vi "save_config.vi"   [LabVIEW 2011]
doc: "Illustrates how to create and write a configuration settings file.\n\nInstructions:\nEnter values in the controls on the front panel then click on the Run Arrow.\nTo read the file, run Read Configuration Settings File.vi located in the file\\config.llb."
uses:
  global.vi
  <vilib>/Utility/config.llb/Write Key (I32).vi
  <vilib>/Utility/config.llb/Write Key (Boolean).vi
  <vilib>/Utility/config.llb/Write Key (Double).vi
  <vilib>/Utility/config.llb/Write Key (String).vi
  <vilib>/Utility/config.llb/NI_LVConfig.lvlib
types:
  T1 = typedef "NI_LVConfig.lvlib/Config Data RefNum.ctl" = refnum<k1>
  T2 = typedef "scale.ctl" = dbl
  T3 = typedef "sampling_rate.ctl" = ext
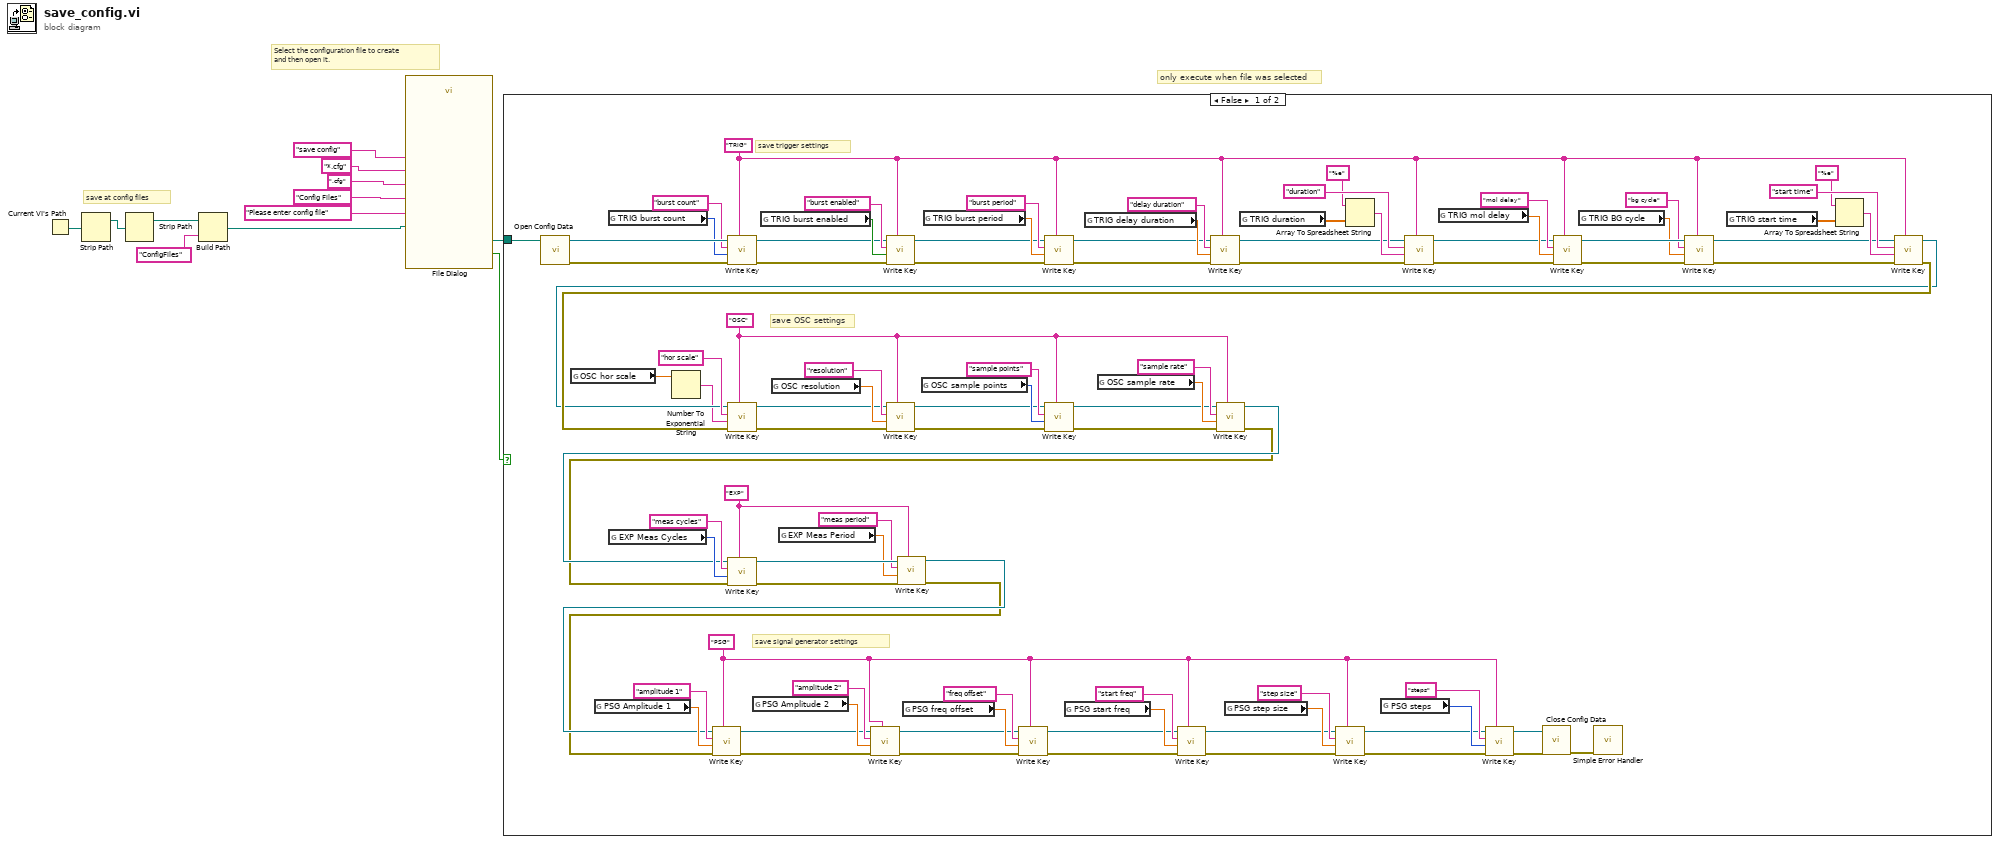
[diagram p0: block diagram]
diagram:
  # "only execute when file was selected"
  # "save at config files"
  # "Select the configuration file to create\nand then open it."
  n1 = Current VI's Path() -> (path=w6:path)
  n2 = Strip Path(path=w6) -> (stripped path=w3:path)  [unwired: 1 out]
  n3 = Strip Path(path=w3) -> (stripped path=w2:path)  [unwired: 1 out]
  n4 = Build Path(base path=w2, name or relative path="ConfigFiles") -> (appended path=w4:path)
  n5 = call "File Dialog"("start path"=w4, "prompt"="Please enter config file", "button label"="save config", "default name"=".cfg", "pattern (all files)"="*.cfg", "pattern label"="Config Files") -> ("selected path"=w12:path, "cancelled"=w1:bool)  [unwired: 6 in, 2 out]
  n6 = case shown="False" w1 {
    tunnel: w12 -> [w101 _]
    frame False {
      w28 = "PSG"
      w19 = "EXP"
      w57 = "OSC"
      w15 = "TRIG"
      # "save signal generator settings"
      # "save OSC settings"
      # "save trigger settings"
      n7 = call <vilib>:"Open Config Data.vi"("configuration file path"=w101) -> ("error out"=w104:errorcluster, "refnum"=w105:T1)  [unwired: 2 in, 7 out]
      n8 = global read "global.vi" "OSC hor scale"() -> (w27:T2)
      n9 = global read "global.vi" "PSG Amplitude 1"() -> (w38:dbl)
      n10 = global read "global.vi" "TRIG burst count"() -> (w100:i32)
      n11 = global read "global.vi" "EXP Meas Cycles"() -> (w55:i32)
      n12 = Number To Exponential String(number=w27) -> (E-format string=w26:string)  [unwired: 3 in]
      n13 = call-poly <vilib>:"Write Key.vi"("section"=w15, "error in (no error)"=w104, "value"=w100, "key"="burst count" ("Key 1"), "refnum"=w105) -> ("error out"=w85:errorcluster, "refnum out"=w89:T1)  [unwired: 5 out]
      n14 = global read "global.vi" "PSG Amplitude 2"() -> (w36:dbl)
      n15 = global read "global.vi" "TRIG burst enabled"() -> (w98:bool)
      n16 = global read "global.vi" "OSC resolution"() -> (w70:ext)
      n17 = global read "global.vi" "EXP Meas Period"() -> (w20:dbl)
      n18 = call-poly <vilib>:"Write Key.vi"("section"=w15, "error in (no error)"=w85, "value"=w98, "key"="burst enabled" ("Key 1"), "refnum"=w89) -> ("error out"=w84:errorcluster, "refnum out"=w88:T1)  [unwired: 5 out]
      n19 = global read "global.vi" "PSG freq offset"() -> (w51:dbl)
      n20 = global read "global.vi" "OSC sample points"() -> (w68:i32)
      n21 = global read "global.vi" "TRIG burst period"() -> (w96:dbl)
      n22 = call-poly <vilib>:"Write Key.vi"("section"=w15, "error in (no error)"=w84, "value"=w96, "key"="burst period" ("Key 1"), "refnum"=w88) -> ("error out"=w83:errorcluster, "refnum out"=w87:T1)  [unwired: 3 in, 2 out]
      n23 = global read "global.vi" "PSG start freq"() -> (w49:dbl)
      n24 = global read "global.vi" "TRIG delay duration"() -> (w94:dbl)
      n25 = global read "global.vi" "OSC sample rate"() -> (w60:T3)
      n26 = call-poly <vilib>:"Write Key.vi"("section"=w15, "error in (no error)"=w83, "value"=w94, "key"="delay duration" ("Key 1"), "refnum"=w87) -> ("error out"=w82:errorcluster, "refnum out"=w86:T1)  [unwired: 3 in, 2 out]
      n27 = global read "global.vi" "PSG step size"() -> (w47:dbl)
      n28 = global read "global.vi" "TRIG duration"() -> (w91:dbl[])
      n29 = Array To Spreadsheet String(array=w91, 3:"%e" ("format string")) -> (spreadsheet string=w90:string)  [unwired: 1 in]
      n30 = global read "global.vi" "PSG steps"() -> (w41:i32)
      n31 = call-poly <vilib>:"Write Key.vi"("section"=w15, "error in (no error)"=w82, "value"=w90, "key"="duration" ("Key 1"), "refnum"=w86) -> ("error out"=w74:errorcluster, "refnum out"=w75:T1)  [unwired: 1 in, 4 out]
      n32 = global read "global.vi" "TRIG mol delay"() -> (w76:dbl)
      n33 = call-poly <vilib>:"Write Key.vi"("section"=w15, "error in (no error)"=w74, "value"=w76, "key"="mol delay" ("Key 1"), "refnum"=w75) -> ("error out"=w73:errorcluster, "refnum out"=w17:T1)  [unwired: 3 in, 2 out]
      n34 = global read "global.vi" "TRIG BG cycle"() -> (w13:dbl)
      n35 = call-poly <vilib>:"Write Key.vi"("section"=w15, "error in (no error)"=w73, "value"=w13, "key"="bg cycle" ("Key 1"), "refnum"=w17) -> ("error out"=w18:errorcluster, "refnum out"=w16:T1)  [unwired: 4 in, 1 out]
      n36 = global read "global.vi" "TRIG start time"() -> (w79:dbl[])
      n37 = Array To Spreadsheet String(array=w79, 3:"%e" ("format string")) -> (spreadsheet string=w78:string)  [unwired: 1 in]
      n38 = call-poly <vilib>:"Write Key.vi"("section"=w15, "error in (no error)"=w18, "value"=w78, "key"="start time" ("Key 1"), "refnum"=w16) -> ("error out"=w63:errorcluster, "refnum out"=w62:T1)  [unwired: 1 in, 4 out]
      n39 = call-poly <vilib>:"Write Key.vi"("section"=w57, "error in (no error)"=w63, "value"=w26, "key"="hor scale" ("Key 1"), "refnum"=w62) -> ("error out"=w65:errorcluster, "refnum out"=w67:T1)  [unwired: 1 in, 4 out]
      n40 = call-poly <vilib>:"Write Key.vi"("section"=w57, "error in (no error)"=w65, "value"=w70, "key"="resolution" ("Key 1"), "refnum"=w67) -> ("error out"=w64:errorcluster, "refnum out"=w66:T1)  [unwired: 3 in, 2 out]
      n41 = call-poly <vilib>:"Write Key.vi"("section"=w57, "error in (no error)"=w64, "value"=w68, "key"="sample points" ("Key 1"), "refnum"=w66) -> ("error out"=w58:errorcluster, "refnum out"=w59:T1)  [unwired: 5 out]
      n42 = call-poly <vilib>:"Write Key.vi"("section"=w57, "error in (no error)"=w58, "value"=w60, "key"="sample rate" ("Key 1"), "refnum"=w59) -> ("error out"=w53:errorcluster, "refnum out"=w54:T1)  [unwired: 3 in, 2 out]
      n43 = call-poly <vilib>:"Write Key.vi"("section"=w19, "error in (no error)"=w53, "value"=w55, "key"="meas cycles" ("Key 1"), "refnum"=w54) -> ("error out"=w24:errorcluster, "refnum out"=w25:T1)  [unwired: 5 out]
      n44 = call-poly <vilib>:"Write Key.vi"("section"=w19, "error in (no error)"=w24, "value"=w20, "key"="meas period" ("Key 1"), "refnum"=w25) -> ("error out"=w22:errorcluster, "refnum out"=w23:T1)  [unwired: 3 in, 2 out]
      n45 = call-poly <vilib>:"Write Key.vi"("section"=w28, "error in (no error)"=w22, "value"=w38, "key"="amplitude 1" ("Key 1"), "refnum"=w23) -> ("error out"=w34:errorcluster, "refnum out"=w35:T1)  [unwired: 3 in, 2 out]
      n46 = call-poly <vilib>:"Write Key.vi"("section"=w28, "error in (no error)"=w34, "value"=w36, "key"="amplitude 2" ("Key 1"), "refnum"=w35) -> ("error out"=w33:errorcluster, "refnum out"=w32:T1)  [unwired: 3 in, 2 out]
      n47 = call-poly <vilib>:"Write Key.vi"("section"=w28, "error in (no error)"=w33, "value"=w51, "key"="freq offset" ("Key 1"), "refnum"=w32) -> ("error out"=w44:errorcluster, "refnum out"=w46:T1)  [unwired: 3 in, 2 out]
      n48 = call-poly <vilib>:"Write Key.vi"("section"=w28, "error in (no error)"=w44, "value"=w49, "key"="start freq" ("Key 1"), "refnum"=w46) -> ("error out"=w43:errorcluster, "refnum out"=w45:T1)  [unwired: 3 in, 2 out]
      n49 = call-poly <vilib>:"Write Key.vi"("section"=w28, "error in (no error)"=w43, "value"=w47, "key"="step size" ("Key 1"), "refnum"=w45) -> ("error out"=w39:errorcluster, "refnum out"=w40:T1)  [unwired: 3 in, 2 out]
      n50 = call-poly <vilib>:"Write Key.vi"("section"=w28, "error in (no error)"=w39, "value"=w41, "key"="steps" ("Key 1"), "refnum"=w40) -> ("error out"=w30:errorcluster, "refnum out"=w31:T1)  [unwired: 5 out]
      n51 = call <vilib>:"Close Config Data.vi"("error in (no error)"=w30, "refnum"=w31) -> ("error out"=w102:errorcluster)  [unwired: 1 in, 8 out]
      n52 = call <vilib>:"Simple Error Handler.vi"("error in (no error)"=w102) -> ()  [unwired: 1 in, 8 out]
    }
    frame True {
    }
  }
